vi "Get String Value Operations.vi"(11 "Operations":T1) -> (3 "Strings[]":string[](array[string]))   [LabVIEW 2016]
uses:
  <vilib>/Utility/miscctls.llb/LVComboBoxStrsAndValuesArrayTypeDef.ctl
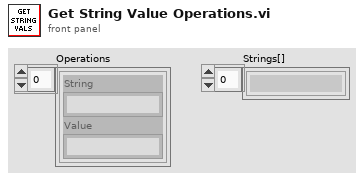
[diagram p1: front panel]
types:
  T1 = typedef "LVComboBoxStrsAndValuesArrayTypeDef.ctl" = cluster{"String":string, "Value":string}[]
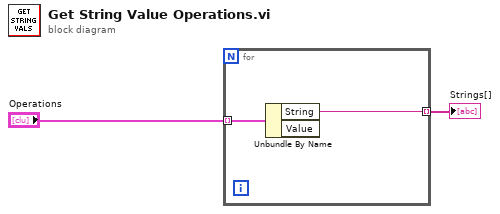
[diagram p0: block diagram]
diagram:
  n1 = for {
    tunnel: "Operations" -> [w4] mode=indexing
    tunnel: [w3] -> w2 mode=indexing
    n2 = Unbundle By Name(w4) -> ("String"=w3:string)  [unwired: 1 out]
  }
  "Strings[]" <- w2
